vi "Find Channel from List.vi"(10 "Aliases.Outputs":T1[](array[typedef]), 11 "Value":string) -> (3 "Channel":T1)   [LabVIEW 2013, in "Simple Sequence Tools - Editor.lvlib"]
uses:
  Simple Sequence Tools - Editor.lvlib
  Shared/Types/Channel.Properties.ctl
  Shared/Simple Sequence Tools - Shared.lvlib
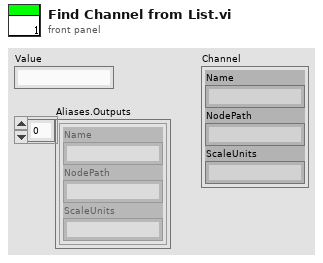
[diagram p1: front panel]
types:
  T1 = typedef "Simple Sequence Tools - Shared.lvlib/Channel.Properties.ctl" = cluster{"Name":string, "NodePath":string, "ScaleUnits":string}
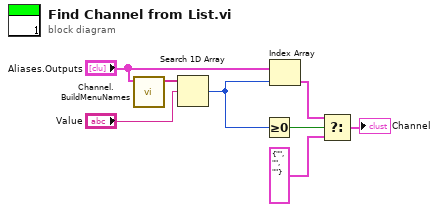
[diagram p0: block diagram]
diagram:
  n1 = call "Channel.BuildMenuNames.vi"("Aliases"="Aliases.Outputs") -> ("Aliases Array"=w6:string[])  [unwired: 10 in]
  n2 = Search 1D Array(1D array=w6, element="Value") -> (index of element=w5:i32)  [unwired: 1 in]
  n3 = Greater Or Equal To 0?(x=w5) -> (x >= 0?=w4:bool)
  n4 = Index Array(array="Aliases.Outputs", index=w5) -> (element=w3:T1)
  n5 = Select(t=w3, s=w4, f=T1 {"Name"="", "NodePath"="", "ScaleUnits"=""} ("Channel")) -> (s? t:f=→"Channel":T1)
